vi "Update Force Bytes.vi"(8 "error in (no error)":errorcluster, 10 "FATypes":T1, 11 "Model in":refnum<class "Model.lvclass">) -> (0 "error out":errorcluster, 3 "Model out":refnum<class "Model.lvclass">)   [LabVIEW 2016]
uses:
  Model.lvclass
  Modbus/DesktopModbus/DesktopModbus.lvclass
  C:/CODE/ts_HPMT/Common_RT_Modbus/IModbus/IModbus.lvclass
  Common_RT_FAILC/DataTypes/HPTypes.ctl
  Common_RT_FAILC/RTHPILC.lvlib
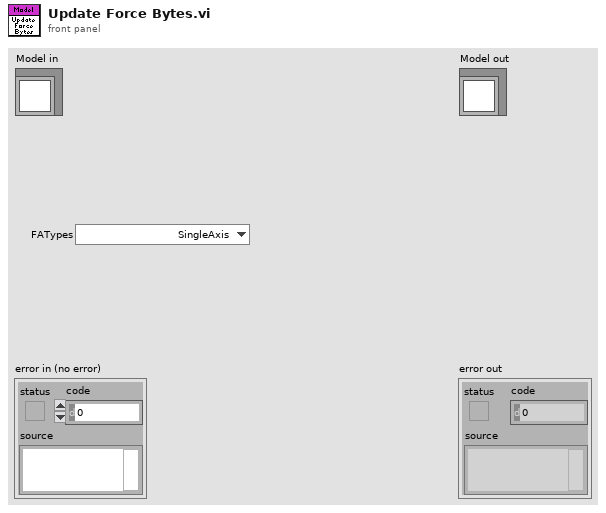
[diagram p1: front panel]
types:
  T1 = typedef "RTHPILC.lvlib/HPTypes.ctl" = enum16{"SingleAxis", "LateralDualAxis", "CrossLateralDualAxis"}
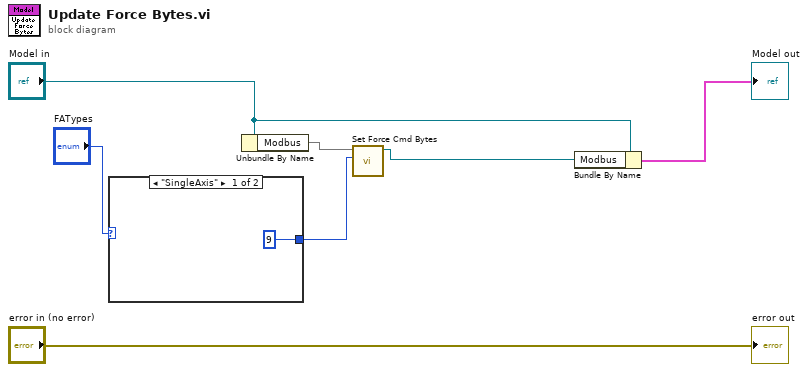
[diagram p0: block diagram]
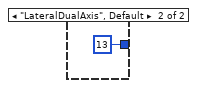
[diagram p2: hidden frame]
diagram:
  n1 = case shown="\"SingleAxis\"" "FATypes" {
    tunnel: [9 13] -> w1
    frame "SingleAxis" {
    }
    frame "LateralDualAxis", Default {
    }
  }
  n2 = Unbundle By Name("Model in") -> ("Modbus"=w7)
  n3 = call "Set Force Cmd Bytes.vi"("ForceCmdBytes"=w1, "DesktopModbus in"=w7) -> ("DesktopModbus out"=w6:refnum<class "DesktopModbus.lvclass">)  [unwired: 9 in]
  n4 = Bundle By Name(cluster="Model in", "Modbus"=w6) -> (→"Model out":cluster{})
  "error out" <- "error in (no error)"
